vi "Code 0.0.6.vi"(0 "Value":refnum<k5>, 1 "status":bool, 3 "File Path Control":path=path "C:/Projects/FlashProgrammer/RayonM1_01.87.01.txt", 5 "Port":u16=8030, 9 "Drv":u8(ring)=1 items=["Drv 1", "Drv 2"], 11 "error in (no error)":errorcluster) -> (4 "Error List":string, 6 "Status":bool, 15 "error out":errorcluster)   [LabVIEW 2017]
panel:
  out "Array":u16[][](array[numeric])
  out "error out 2":errorcluster
  in  "Delay between sub packets":dbl=0.01 format="%#_13g"
  in  "sub packet Data Length":i32=64
  in  "stop":bool
  out "Time Elapsed":dbl
  in  "MaxSlide":dbl
  out "Autobaud":bool
  in  "StopS.M. 2":bool
  in  "StopS.M.":bool
  in  "CatchNetworkFlag":bool
  in  "stop Listen":bool
  out "conn ID":refnum<k5>
  in  "Next Button":bool
  out "CheckSum":bool[][](array[boolean])
  out "CheckSum DataB":u16 format="%.0x"
  out "CheckSum Data":u16 format="%.0x"
  out "Writting Data":bool
  out "Send Header":bool
  out "sumHeader":u16 format="%.0x"
  # "Ver 0.0.7"
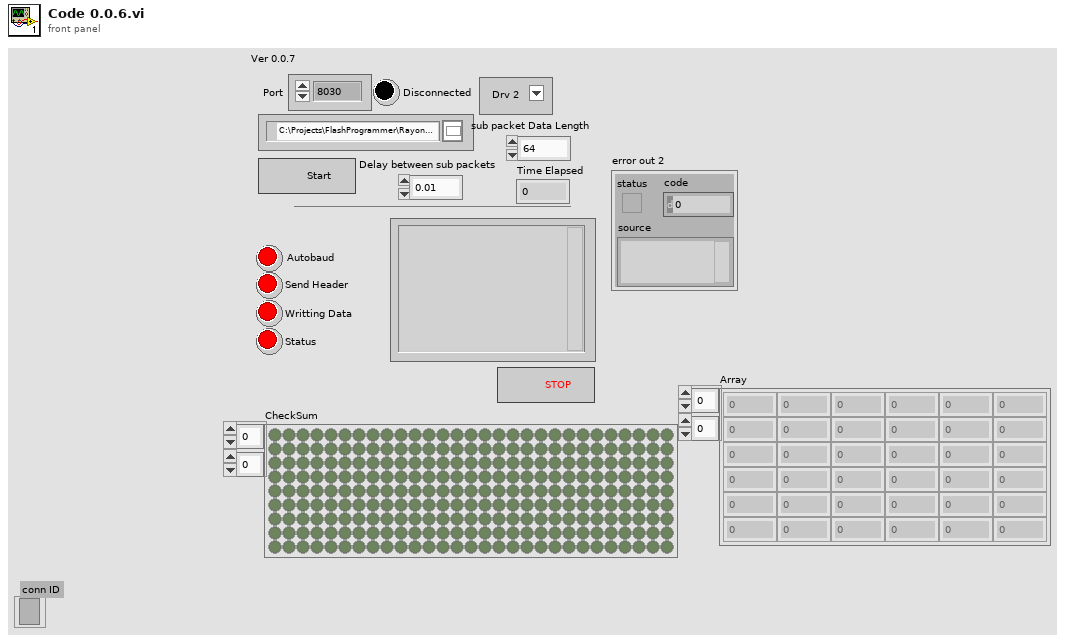
[diagram p1: front panel]
types:
  T1 = enum16{"open", "replace", "create", "open or create", "replace or create", "replace or create with confirmation"}
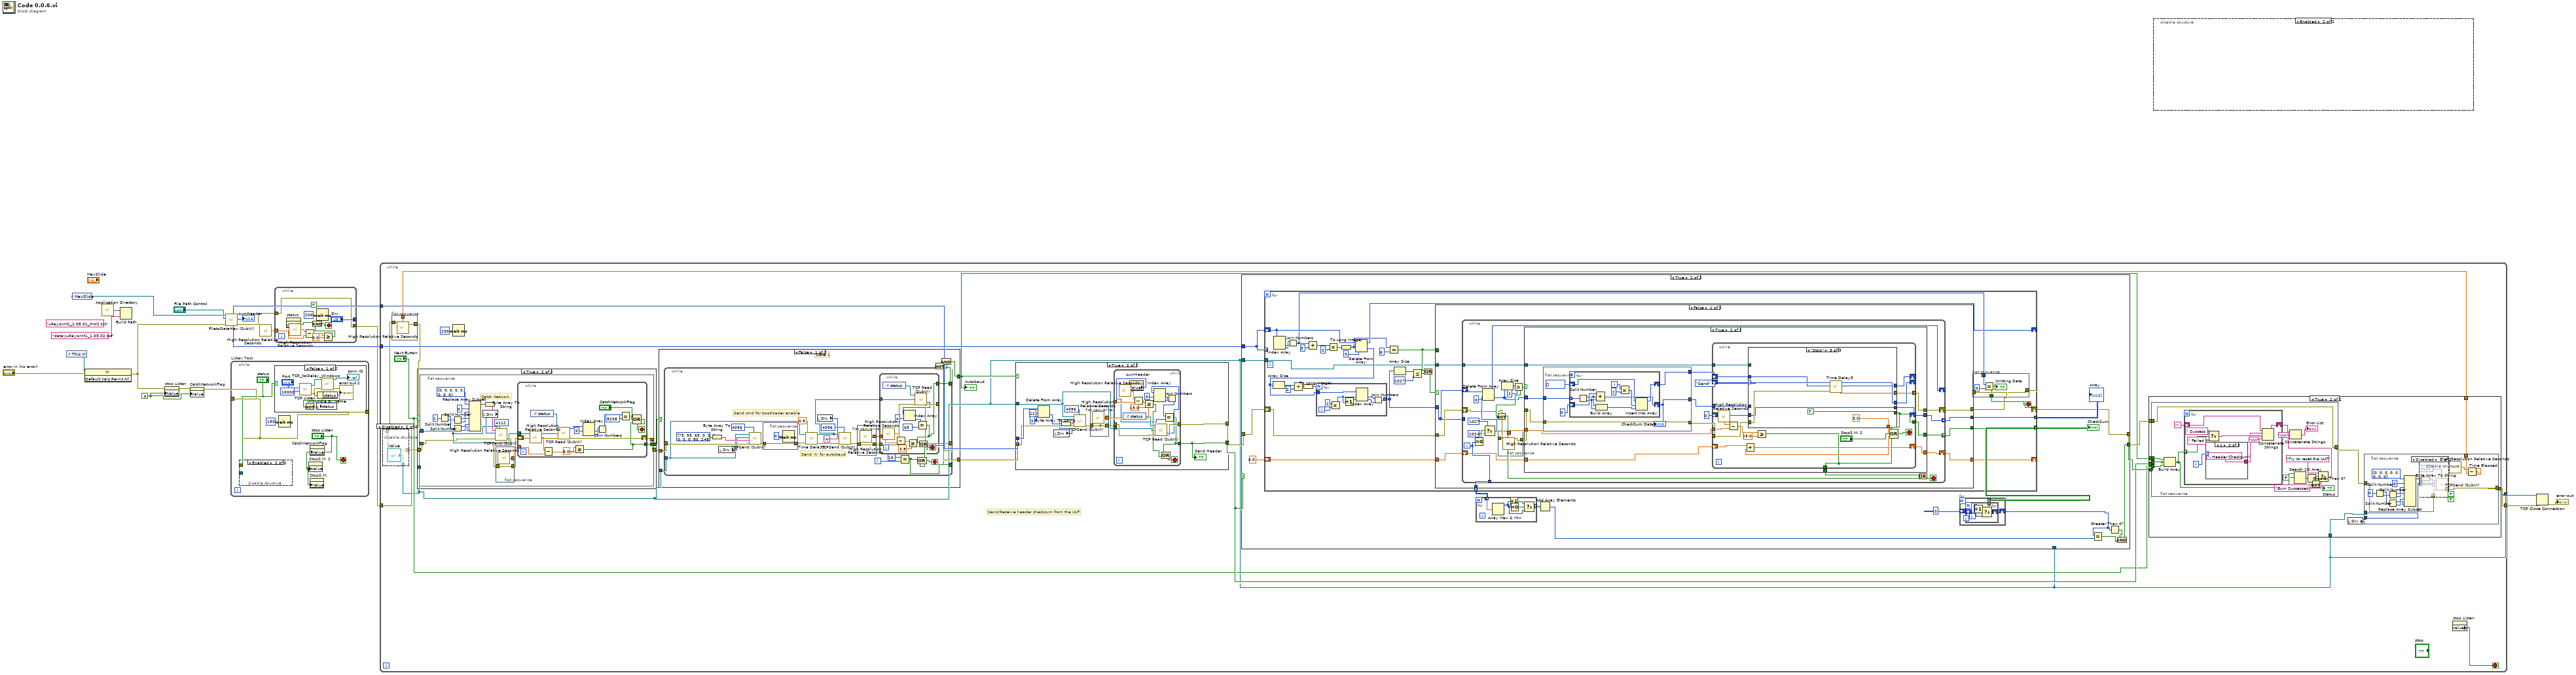
[diagram p0: block diagram]
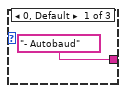
[diagram p4: hidden frame]
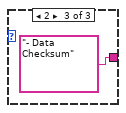
[diagram p5: hidden frame]
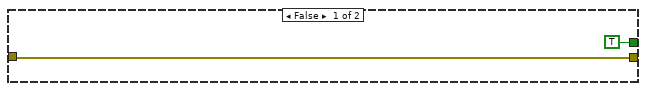
[diagram p6: hidden frame]
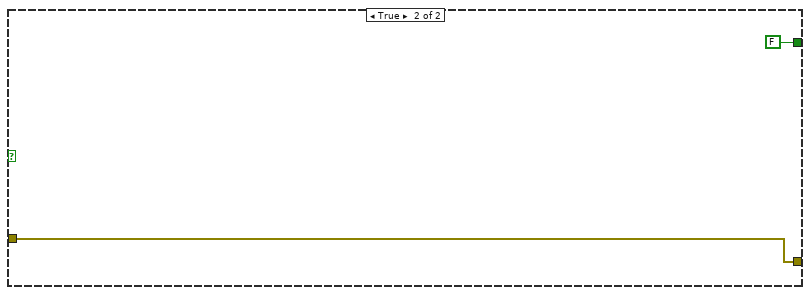
[diagram p7: hidden frame]
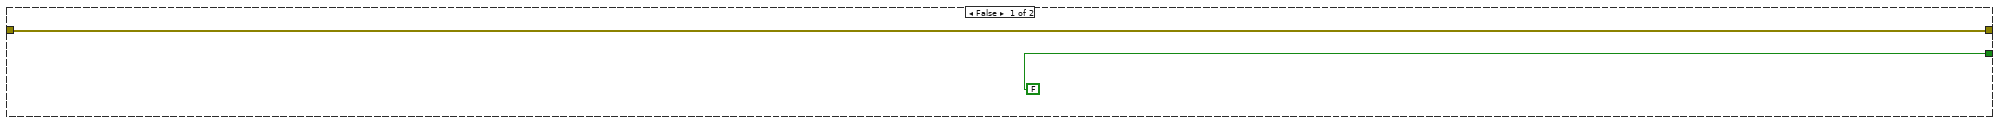
[diagram p8: hidden frame]
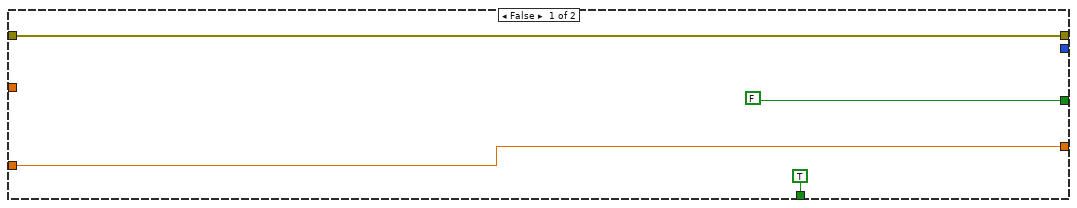
[diagram p9: hidden frame]
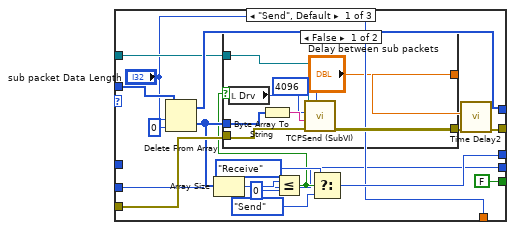
[diagram p10: hidden frame]
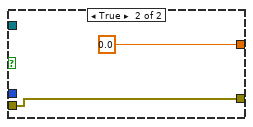
[diagram p11: hidden frame]
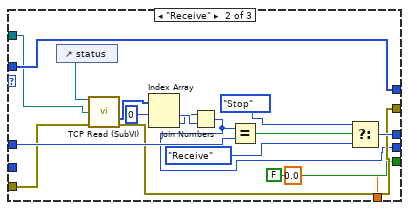
[diagram p12: hidden frame]
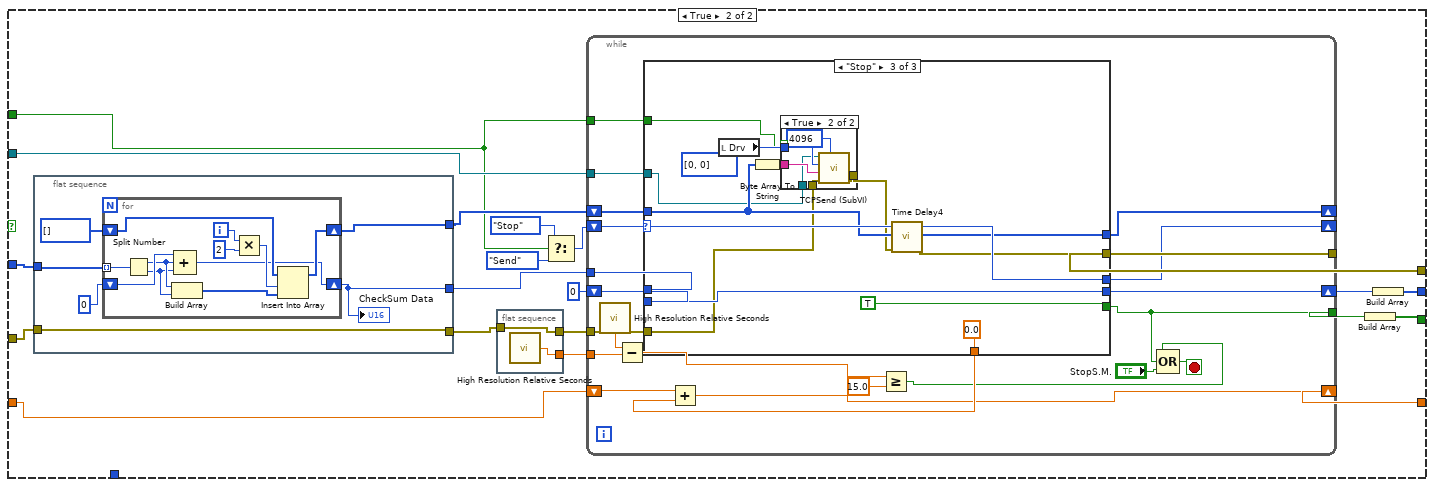
[diagram p13: hidden frame]
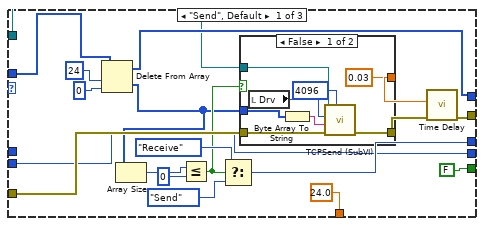
[diagram p14: hidden frame]
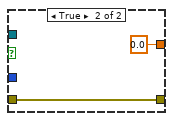
[diagram p15: hidden frame]
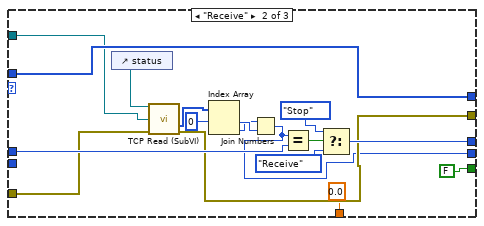
[diagram p16: hidden frame]
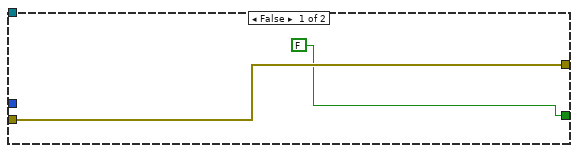
[diagram p18: hidden frame]
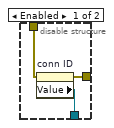
[diagram p19: hidden frame]
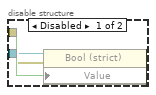
[diagram p20: hidden frame]
diagram:
  (unwired) "uRayonM1_1.05.01_HW2.txt" ("name or relative path")
  w7 = FALSE ("stop")
  n1 = control-ref of="This VI"() -> (w5:refnum<vi>)
  n2 = control-ref of="MaxSlide"() -> (w6:refnum<vi>)
  n3 = invoke class="VI" method="Default Vals.Reinit All"(reference=w5, error in="error in (no error)") -> (error out=w9:errorcluster)  [unwired: 1 in, 2 out]
  n4 = call <vilib>:"Application Directory.vi"() -> ("Application Directory"=w13:path)
  n5 = Build Path(base path=w13, name or relative path="data\\uRayonM1_1.03.02.txt") -> ()  [unwired: 1 out]
  n6 = property on="stop Listen" class="Bool (strict)"(error in=w9, "Value"=w7) -> (error out=w8:errorcluster)  [unwired: 1 in, 1 out]
  n7 = property on="CatchNetworkFlag" class="Bool (strict)"(error in=w8, "Value"=w7) -> (error out=w12:errorcluster)  [unwired: 1 in, 1 out]
  n8 = call "FiletoDataHex (SubVI).vi"("error constant"=w9, "file path (use dialog)"="File Path Control", "Progress bar Max"=w6) -> ("error constant 2"=w4:errorcluster, "Array 2"=w19:u8[], "Array"=w17:u8[], "sumHeader"=→"sumHeader":u16)  [unwired: 2 in, 3 out]
  n9 = while "Listen Task" {
    tunnel: w12 -> [w21]
    tunnel: [w21] -> _
    stop <- "stop Listen" stop-if-true
    n10 = disable-structure shown="Enabled" {
      disable-tunnel: "status" -> [w26 _]
      disable-tunnel: w21 -> [w25 _]
      disable-tunnel: _ -> [w24 _]
      frame Disabled {
        n11 = property class="Bool (strict)"(reference=w24, error in=w25, "Value"=w26) -> ()  [unwired: 2 out]
      }
      frame Enabled {
      }
    }
    n12 = case shown="False" "status" {
      selector: "status" -> [_ w35]
      frame False {
        n13 = call <vilib>:"TCP Listen.vi"("timeout ms (wait forever: -1)"=10000, "port"="Port") -> ("error out"=w28:errorcluster, "connection ID"=w30:refnum<k5>)  [unwired: 5 in, 3 out]
        n14 = Unbundle By Name(w28) -> ("status"=w31:bool)
        n15 = Not(x=w31) -> (.not. x?=w32:bool)
        n16 = local write "status"(w32) -> ()
        n17 = call "TCP_NoDelay_Windows.vi"("error in (no error)"=w28, "connID"=w30) -> ("error out"=→"error out 2":errorcluster, "connID 2"=→"conn ID":refnum<k5>)  [unwired: 4 in]
      }
      frame True {
        n18 = property on="status" class="Bool (strict)"("Value"=w35) -> ()  [unwired: 2 in, 2 out]
      }
    }
    n19 = Wait (ms)(milliseconds to wait=u32 150) -> ()  [unwired: 1 out]
    n20 = property on="StopS.M. 2" class="Bool (strict)"("Value"="stop Listen") -> ()  [unwired: 2 in, 2 out]
    n21 = property on="StopS.M." class="Bool (strict)"("Value"="stop Listen") -> ()  [unwired: 2 in, 2 out]
    n22 = property on="CatchNetworkFlag" class="Bool (strict)"("Value"="stop Listen") -> ()  [unwired: 2 in, 2 out]
  }
  n23 = call <vilib>:"High Resolution Relative Seconds.vi"() -> ("relative seconds"=w11:dbl)
  n24 = while {
    tunnel: w4 -> [w43]
    tunnel: ["Drv"] -> _
    tunnel: [w43] -> w2
    tunnel: w11 -> [w41]
    stop <- w38 stop-if-true
    (unwired) TRUE
    n25 = property on="status" class="Bool (strict)"() -> ("Value"=w36:bool)  [unwired: 2 in, 2 out]
    n26 = call <vilib>:"High Resolution Relative Seconds.vi"() -> ("relative seconds"=w42:dbl)
    n27 = Subtract(x=w42, y=w41) -> (x-y=w40:dbl)
    n28 = Wait (ms)(milliseconds to wait=u32 200) -> ()  [unwired: 1 out]
    n29 = Greater Or Equal?(x=w40, y=3.0) -> (x >= y?=w37:bool)
    n30 = And(x=w36, y=w37) -> (x .and. y?=w38:bool)
  }
  n31 = while {
    tunnel: w19 -> [w64]
    tunnel: w17 -> [w61]
    tunnel: [w46] -> w3
    tunnel: w2 -> [w52]
    tunnel: [w58] -> w16
    stop <- w49 stop-if-true
    # "Send/Receive header checksum from the UUT"
    n32 = disable-structure shown="Disabled" {
      disable-tunnel: w51 -> [w607 w609]
      disable-tunnel: [w606 w609] -> w54
      disable-tunnel: [w605 "Value"] -> w46
      frame Enabled {
        n33 = property on="conn ID" class="Ref (strict)"(error in=w607) -> (error out=w606:errorcluster, "Value"=w605:refnum<k5>)  [unwired: 1 in, 1 out]
      }
      frame Disabled {
      }
    }
    n34 = flat-sequence {
      tunnel: w52 -> [w174]
      tunnel: [w174] -> _
      tunnel: [w175] -> w50
      tunnel: [w174] -> w51
      frame #0 {
        n35 = call <vilib>:"High Resolution Relative Seconds.vi"() -> ("relative seconds"=w175:dbl)
      }
    }
    n36 = case shown="True" "Next Button" {
      tunnel: [w129 w133] -> w62
      tunnel: w54 -> [w129 w132]
      tunnel: w46 -> [_ w131]
      tunnel: [TRUE ("Time has Elapsed") w130] -> w53
      frame False {
      }
      frame True {
        n37 = flat-sequence {
          tunnel: w131 -> [w139]
          tunnel: [w141] -> w133
          tunnel: w132 -> [w137]
          tunnel: [w138] -> w130
          frame #0 {
            # "Catch Network"
            n38 = Split Number(x=u32 1) -> (hi(x)=w151:u16, lo(x)=w150:u16)
            n39 = Split Number(x=w150) -> (hi(x)=w145:u8, lo(x)=w144:u8)
            n40 = Split Number(x=w151) -> (hi(x)=w143:u8, lo(x)=w142:u8)
            n41 = Replace Array Subset(array=u8[] [0, 0, 0, 0, 0, 0, 0, 0] ("unsigned byte array"), new element #1=w144, index #1=0 ("index"), new element #2=w145, new element #3=w142, new element #4=w143) -> (w146:u8[])  [unwired: 3 in]
            n42 = local read "Drv"() -> (w140:u8)
            n43 = Byte Array To String(unsigned byte array=w146) -> (string=w152:string)
            n44 = call "TCPSend (SubVI).vi"("Opcode"=u32 4112, "error in"=w137, "string"=w152, "Drv"=w140, "connection ID"=w139) -> ("error out"=w134:errorcluster)  [unwired: 6 in]
            n45 = flat-sequence {
              tunnel: w134 -> [w154]
              tunnel: [w155] -> w135
              tunnel: [w154] -> w136
              frame #0 {
                n46 = call <vilib>:"High Resolution Relative Seconds.vi"() -> ("relative seconds"=w155:dbl)
              }
            }
            n47 = while {
              shift-right: [w172] -> w141
              shift-left: w136 -> [w173]
              tunnel: w139 -> [w161]
              tunnel: [w156] -> w138
              tunnel: w135 -> [w159]
              stop <- w167 stop-if-true
              n48 = call <vilib>:"High Resolution Relative Seconds.vi"() -> ("relative seconds"=w160:dbl)
              n49 = control-ref of="status"() -> (w166:refnum<vi>)
              n50 = Subtract(x=w160, y=w159) -> (x-y=w158:dbl)
              n51 = call "TCP Read (SubVI).vi"("Status in"=w166, "Value"=w161, "error in (no error)"=w173) -> ("Rx data tmp"=w165:u8[], "error out"=w172:errorcluster)  [unwired: 2 in, 9 out]
              n52 = Greater Or Equal?(x=w158, y=5.0) -> (x >= y?=w156:bool)
              n53 = Index Array(array=w165, index #1=0 ("index")) -> (element #1=w164:u8, element #2=w163:u8)  [unwired: 1 in]
              n54 = Join Numbers(hi=w163, lo=w164) -> ((hi.lo)=w171:u16)
              n55 = Equal?(x=w171, y=u16 8208) -> (x = y?=w169:bool)
              n56 = Compound Arithmetic op=OR("CatchNetworkFlag", w169, w156) -> (w167:bool)
            }
          }
        }
      }
    }
    n57 = Wait (ms)(milliseconds to wait=u32 200) -> ()  [unwired: 1 out]
    n58 = case shown="False" w53 {
      tunnel: w62 -> [w182 w224]
      tunnel: [w181 w224] -> w59
      tunnel: [w179 FALSE] -> w55
      tunnel: w46 -> [w180 _]
      frame False {
        # "State 1"
        n59 = while {
          tunnel: w182 -> [w199]
          tunnel: [w197] -> w181
          tunnel: w180 -> [w184]
          tunnel: [w187] -> w178
          tunnel: [w183] -> w177
          i -> [w203]
          stop <- w204 stop-if-true
          # "Send 'A' for autobaud"
          # "Send cmd for bootloader enable"
          n60 = Byte Array To String(unsigned byte array=u8[] [73, 93, 65, 0, 0, 1, 0, 0, 0, 80, 248] ("output array")) -> (string=w193:string)
          n61 = local read "Drv"() -> (w188:u8)
          n62 = call "TCPSend (SubVI).vi"("Opcode"=u32 4096, "error in"=w199, "string"=w193, "Drv"=w188, "connection ID"=w184) -> ("error out"=w195:errorcluster)  [unwired: 6 in]
          n63 = flat-sequence {
            tunnel: w195 -> [w205]
            tunnel: [w205] -> w194
            frame #0 {
              n64 = Wait (ms)(milliseconds to wait=u32 0) -> ()  [unwired: 1 out]
            }
          }
          n65 = call "Time Delay3"("error in (no error)"=w194, "Delay Time (s)"=0.5) -> ("error out"=w186:errorcluster)  [unwired: 9 in]
          n66 = local read "Drv"() -> (w189:u8)
          n67 = call "TCPSend (SubVI).vi"("Opcode"=u32 4096, "error in"=w186, "string"="A" ("write buffer"), "Drv"=w189, "connection ID"=w184) -> ("error out"=w198:errorcluster)  [unwired: 6 in]
          n68 = flat-sequence {
            tunnel: w198 -> [w208]
            tunnel: [w208] -> w201
            tunnel: [w207] -> w200
            frame #0 {
              n69 = call <vilib>:"High Resolution Relative Seconds.vi"() -> ("relative seconds"=w207:dbl)
            }
          }
          n70 = while {
            tunnel: w201 -> [w213]
            tunnel: w200 -> [w219]
            tunnel: [w212] -> w197
            tunnel: [w210] -> w187
            tunnel: w184 -> [w209]
            stop <- w211 stop-if-true
            n71 = control-ref of="status"() -> (w223:refnum<vi>)
            n72 = call <vilib>:"High Resolution Relative Seconds.vi"() -> ("relative seconds"=w220:dbl)
            n73 = Subtract(x=w220, y=w219) -> (x-y=w218:dbl)
            n74 = Greater Or Equal?(x=w218, y=0.5) -> (x >= y?=w216:bool)
            n75 = call "TCP Read (SubVI).vi"("Status in"=w223, "Value"=w209, "error in (no error)"=w213) -> ("Drv Array"=w221:u8[], "error out"=w212:errorcluster)  [unwired: 2 in, 9 out]
            n76 = Index Array(array=w221, index=0) -> (element=w215:u8)
            n77 = Equal?(x=w215, y=u8 65) -> (x = y?=w210:bool)
            n78 = Or(x=w210, y=w216) -> (x .or. y?=w211:bool)
          }
          n79 = Equal?(x=10, y=w203) -> (x = y?=w183:bool)
          n80 = Compound Arithmetic op=OR(w183, w187) -> (w204:bool)
        }
        n81 = Not(x=w177) -> (.not. x?=w176:bool)
        n82 = And(x=w178, y=w176) -> (x .and. y?=w179:bool)
      }
      frame True {
      }
    }
    "Autobaud" <- w55
    n83 = case shown="True" w55 {
      tunnel: w59 -> [w571 w583]
      tunnel: [w571 w585] -> w57
      tunnel: w61 -> [_ w584]
      tunnel: [FALSE w574] -> w56
      tunnel: w46 -> [_ w572]
      frame False {
      }
      frame True {
        n84 = Delete From Array(array=w584, length=22, index=0) -> (deleted portion=w579:u8[])  [unwired: 1 out]
        n85 = local read "Drv"() -> (w573:u8)
        n86 = Byte Array To String(unsigned byte array=w579) -> (string=w577:string)
        n87 = call "TCPSend (SubVI).vi"("Opcode"=u32 4096, "error in"=w583, "string"=w577, "Drv"=w573, "connection ID"=w572) -> ("error out"=w582:errorcluster)  [unwired: 6 in]
        n88 = flat-sequence {
          tunnel: w582 -> [w586]
          tunnel: [w586] -> _
          tunnel: [w587] -> w575
          tunnel: [w586] -> w576
          frame #0 {
            n89 = call <vilib>:"High Resolution Relative Seconds.vi"() -> ("relative seconds"=w587:dbl)
          }
        }
        n90 = while {
          tunnel: w576 -> [w599]
          tunnel: [w598] -> w585
          tunnel: w575 -> [w603]
          tunnel: [w589] -> w574
          tunnel: w572 -> [w588]
          stop <- w595 stop-if-true
          n91 = call <vilib>:"High Resolution Relative Seconds.vi"() -> ("relative seconds"=w604:dbl)
          n92 = control-ref of="status"() -> (w600:refnum<vi>)
          n93 = property on="sumHeader" class="DigNum (strict)"() -> ("Value"=w590:u16)  [unwired: 2 in, 2 out]
          n94 = Subtract(x=w604, y=w603) -> (x-y=w602:dbl)
          n95 = Greater Or Equal?(x=w602, y=15.0) -> (x >= y?=w594:bool)
          n96 = call "TCP Read (SubVI).vi"("Status in"=w600, "Value"=w588, "error in (no error)"=w599) -> ("Drv Array"=w596:u8[], "error out"=w598:errorcluster)  [unwired: 2 in, 9 out]
          n97 = Index Array(array=w596, index #1=0 ("index")) -> (element #1=w592:u8, element #2=w593:u8)  [unwired: 1 in]
          n98 = Join Numbers(hi=w593, lo=w592) -> ((hi.lo)=w591:u16)
          n99 = Equal?(x=w591, y=w590) -> (x = y?=w589:bool)
          n100 = Compound Arithmetic op=OR(w589, w594) -> (w595:bool)
        }
        "Send Header" <- w574
      }
    }
    n101 = case shown="True" w56 {
      tunnel: w57 -> [w226 w241]
      tunnel: [w226 w228] -> w60
      tunnel: w64 -> [_ w242]
      tunnel: [FALSE w232] -> w63
      tunnel: w46 -> [_ w231]
      tunnel: w46 -> [_ _]
      frame False {
      }
      frame True {
        n102 = for {
          shift-right: [w279] -> _
          shift-left: w242 -> [w287]
          tunnel: w242 -> [_] mode=indexing
          tunnel: [w268] -> w238 mode=indexing
          shift-right: [w255] -> w228
          shift-left: w241 -> [w264]
          tunnel: [w263] -> w240 mode=indexing
          tunnel: w231 -> [w262]
          shift-right: [w260] -> _
          shift-left: 0.0 -> [w261]
          tunnel: [w259] -> w229 mode=indexing
          stop <- w257 stop-if-true
          n103 = Index Array(array=w287) -> (element #1=w286:u8, element #2=w285:u8)  [unwired: 2 in]
          n104 = Join Numbers(hi=w285, lo=w286) -> ((hi.lo)=w258:u16)
          n105 = Add(x=w258, y=u32 3) -> (x+y=w283:u32)
          n106 = Multiply(x=w283, y=u32 2) -> (x*y=w281:u32)
          n107 = To Long Integer(number=w281) -> (32bit integer=w266:i32)
          n108 = Delete From Array(array=w287, length=w266, index=0) -> (deleted portion=w267:u8[], array with subset deleted=w279:u8[])
          n109 = Array Size(array=w267) -> (size(s)=w276:i32)
          n110 = Divide(x=w276, y=2) -> (x/y=w278:dbl)
          n111 = To Long Integer(number=w278) -> (32bit integer=w275:i32)
          n112 = for {
            N: w275 -> [_]
            tunnel: w267 -> [w566]
            tunnel: [w562] -> w272 mode=indexing
            i -> [w565]
            n113 = Multiply(x=2, y=w565) -> (x*y=w568:i32)
            n114 = Increment(x=w568) -> (x+1=w569:i32)
            n115 = Index Array(array=w566, index #1=w568, index #2=w569) -> (element #1=w564:u8, element #2=w563:u8)
            n116 = Join Numbers(hi=w564, lo=w563) -> ((hi.lo)=w562:u16)
          }
          n117 = Equal?(x=w266, y=6) -> (x = y?=w265:bool)
          n118 = Array Size(array=w272) -> (size(s)=w274:i32)
          n119 = Less Or Equal?(x=w274, y=1027) -> (x <= y?=w270:bool)
          n120 = Or(x=w265, y=w270) -> (x .or. y?=w269:bool)
          n121 = case shown="False" w269 {
            tunnel: w264 -> [w299 w453]
            tunnel: [w300 w451] -> w256
            tunnel: w272 -> [w297 w455]
            tunnel: [w298 w454] -> w268
            tunnel: w265 -> [_ w436]
            tunnel: [w296 _] -> w263
            tunnel: w262 -> [w295 w445]
            tunnel: w261 -> [w294 w444]
            tunnel: [w293 w443] -> w260
            tunnel: [w292 w438] -> w259
            frame False {
              n122 = while {
                tunnel: w297 -> [_]
                tunnel: [w312] -> w298 mode=indexing
                shift-right: [w324] -> w300
                shift-left: w299 -> [w303]
                shift-right: [w317] -> _
                shift-left: w297 -> [w323]
                tunnel: [w310] -> w296 mode=indexing
                tunnel: w295 -> [w309]
                shift-right: [w307] -> w293
                shift-left: w294 -> [w308]
                tunnel: [w301] -> w292 mode=indexing
                i -> [w310]
                stop <- w306 stop-if-true
                n123 = Equal To 0?(x=w310) -> (x = 0?=w316:bool)
                n124 = Select(t=1027 ("length"), s=w316, f=1024 ("length")) -> (s? t:f=w313:i32)
                n125 = Delete From Array(array=w323, length=w313, index=0) -> (deleted portion=w311:u16[], array with subset deleted=w317:u16[])
                n126 = flat-sequence {
                  tunnel: w303 -> [w326]
                  tunnel: [w326] -> w302
                  tunnel: [w325] -> w304
                  frame #0 {
                    n127 = call <vilib>:"High Resolution Relative Seconds.vi"() -> ("relative seconds"=w325:dbl)
                  }
                }
                n128 = Array Size(array=w311) -> (size(s)=w321:i32)
                n129 = Greater?(x=w321, y=1) -> (0:w319:bool)
                n130 = Not(x=w319) -> (.not. x?=w318:bool)
                n131 = case shown="True" w319 {
                  tunnel: [w330 w342] -> w324
                  tunnel: w302 -> [w330 w344]
                  tunnel: [FALSE w340] -> w312
                  tunnel: w311 -> [_ w345]
                  tunnel: w309 -> [_ w338]
                  tunnel: w308 -> [w328 w337]
                  tunnel: [w328 w336] -> w307
                  tunnel: [TRUE ("Time has Elapsed") w335] -> w305
                  tunnel: w304 -> [_ w334]
                  tunnel: [_ w332] -> w301
                  frame False {
                  }
                  frame True {
                    n132 = flat-sequence {
                      tunnel: w344 -> [w420]
                      tunnel: [w422] -> w339
                      tunnel: [w419] -> w341
                      tunnel: w345 -> [w421]
                      tunnel: [w420] -> w333
                      frame #0 {
                        n133 = for {
                          tunnel: w421 -> [w435] mode=indexing
                          shift-right: [w430] -> w422
                          shift-left: u8[] [] -> [w429]
                          shift-right: [w427] -> w419
                          shift-left: u16 0 -> [w428]
                          i -> [w434]
                          n134 = Split Number(x=w435) -> (hi(x)=w426:u8, lo(x)=w425:u8)
                          n135 = Build Array(w426, w425) -> (w432:u8[])
                          n136 = Compound Arithmetic op=ADD(w428, w426, w425) -> (w427:u16)
                          n137 = Multiply(x=w434, y=2) -> (x*y=w431:i32)
                          n138 = Insert Into Array(array=w429, index=w431, new element=w432) -> (w430:u8[])
                        }
                        "CheckSum DataB" <- w419
                      }
                    }
                    n139 = while {
                      shift-right: [w364] -> _
                      shift-left: enum16{"Stop", "Receive", "Send"}."Send" -> [w366]
                      shift-right: [w362] -> _
                      shift-left: w339 -> [w365]
                      tunnel: w341 -> [w363]
                      tunnel: [w358] -> w340
                      tunnel: [w361] -> w342
                      tunnel: w338 -> [w357]
                      shift-right: [w354] -> w336
                      shift-left: w337 -> [w356]
                      tunnel: [w349] -> w335
                      tunnel: w333 -> [w353]
                      tunnel: w334 -> [w348]
                      shift-right: [w347] -> w332
                      shift-left: u16 0 -> [w346]
                      stop <- w360 stop-if-true
                      n140 = call <vilib>:"High Resolution Relative Seconds.vi"() -> ("relative seconds"=w352:dbl)
                      n141 = Subtract(x=w352, y=w348) -> (x-y=w351:dbl)
                      n142 = case shown="\"Stop\"" w366 {
                        selector: w366 -> [_ _ w418]
                        tunnel: w365 -> [w383 w402 w416]
                        tunnel: [w380 w404 w418] -> w364
                        tunnel: w353 -> [w379 w400 w415]
                        tunnel: w363 -> [_ w406 _]
                        tunnel: [FALSE FALSE TRUE] -> w358
                        tunnel: [w375 w402 w416] -> w362
                        tunnel: [w373 w401 w412] -> w361
                        tunnel: w357 -> [w369 w397 _]
                        tunnel: ["sub packet Data Length" 0.0 ("y") 0.0 ("y")] -> w355
                        tunnel: [w367 w395 w413] -> w347
                        tunnel: w346 -> [w367 _ w413]
                        frame "Send", Default {
                          n143 = Delete From Array(array=w383, length="sub packet Data Length", index=0) -> (deleted portion=w372:u8[], array with subset deleted=w375:u8[])
                          n144 = Array Size(array=w372) -> (size(s)=w381:i32)
                          n145 = Less Or Equal?(x=w381, y=0) -> (x <= y?=w371:bool)
                          n146 = case shown="False" w371 {
                            tunnel: w372 -> [w389 _]
                            tunnel: w379 -> [w388 w394]
                            tunnel: [w387 w394] -> w374
                            tunnel: ["Delay between sub packets" 0.0 ("Delay Time (s)")] -> w370
                            tunnel: w369 -> [w385 _]
                            frame False {
                              n147 = local read "Drv"() -> (w390:u8)
                              n148 = Byte Array To String(unsigned byte array=w389) -> (string=w391:string)
                              n149 = call "TCPSend (SubVI).vi"("Opcode"=u32 4096, "error in"=w388, "string"=w391, "Drv"=w390, "connection ID"=w385) -> ("error out"=w387:errorcluster)  [unwired: 6 in]
                            }
                            frame True {
                            }
                          }
                          n150 = Select(t=enum16{"Stop", "Receive", "Send"}."Receive", s=w371, f=enum16{"Stop", "Receive", "Send"}."Send") -> (s? t:f=w380:enum16{"Stop", "Receive", "Send"})
                          n151 = call "Time Delay2"("error in (no error)"=w374, "Delay Time (s)"=w370) -> ("error out"=w373:errorcluster)  [unwired: 9 in]
                        }
                        frame "Receive" {
                          n152 = control-ref of="status"() -> (w411:refnum<vi>)
                          n153 = call "TCP Read (SubVI).vi"("Status in"=w411, "Value"=w397, "error in (no error)"=w400) -> ("Drv Array"=w407:u8[], "error out"=w401:errorcluster)  [unwired: 2 in, 9 out]
                          n154 = Index Array(array=w407, index #1=0 ("index")) -> (element #1=w410:u8, element #2=w409:u8)  [unwired: 1 in]
                          n155 = Join Numbers(hi=w409, lo=w410) -> ((hi.lo)=w395:u16)
                          n156 = Equal?(x=w395, y=w406) -> (x = y?=w399:bool)
                          n157 = Select(t=enum16{"Stop", "Receive", "Send"}."Stop", s=w399, f=enum16{"Stop", "Receive", "Send"}."Receive") -> (s? t:f=w404:enum16{"Stop", "Receive", "Send"})
                        }
                        frame "Stop" {
                          n158 = call "Time Delay5"("error in (no error)"=w415) -> ("error out"=w412:errorcluster)  [unwired: 10 in]
                        }
                      }
                      n159 = Add(x=w356, y=w355) -> (x+y=w354:dbl)
                      n160 = Greater Or Equal?(x=w351, y=15.0) -> (x >= y?=w349:bool)
                      n161 = Compound Arithmetic op=OR(w358, "StopS.M. 2", w349) -> (w360:bool)
                    }
                  }
                }
                n162 = Or(x=w305, y=w318) -> (x .or. y?=w306:bool)
              }
            }
            frame True {
              n163 = flat-sequence {
                tunnel: w453 -> [w546]
                tunnel: [w548] -> w446
                tunnel: w455 -> [w547]
                tunnel: [w546] -> w442
                tunnel: [w545] -> w452
                frame #0 {
                  n164 = for {
                    tunnel: w547 -> [w561] mode=indexing
                    shift-right: [w556] -> w548
                    shift-left: u8[] [] -> [w555]
                    shift-right: [w553] -> w545
                    shift-left: u16 0 -> [w554]
                    i -> [w560]
                    n165 = Split Number(x=w561) -> (hi(x)=w552:u8, lo(x)=w551:u8)
                    n166 = Build Array(w552, w551) -> (w558:u8[])
                    n167 = Compound Arithmetic op=ADD(w554, w552, w551) -> (w553:u16)
                    n168 = Multiply(x=w560, y=2) -> (x*y=w557:i32)
                    n169 = Insert Into Array(array=w555, index=w557, new element=w558) -> (w556:u8[])
                  }
                  "CheckSum Data" <- w545
                }
              }
              n170 = flat-sequence {
                tunnel: w442 -> [w457]
                tunnel: [w457] -> w441
                tunnel: [w456] -> w440
                frame #0 {
                  n171 = call <vilib>:"High Resolution Relative Seconds.vi"() -> ("relative seconds"=w456:dbl)
                }
              }
              n172 = Select(t=enum16{"Stop", "Receive", "Send"}."Stop", s=w436, f=enum16{"Stop", "Receive", "Send"}."Send") -> (s? t:f=w449:enum16{"Stop", "Receive", "Send"})
              n173 = while {
                shift-right: [w477] -> _
                shift-left: w449 -> [w479]
                shift-right: [w475] -> _
                shift-left: w446 -> [w478]
                tunnel: w441 -> [w468]
                tunnel: w452 -> [w476]
                tunnel: [w474] -> w447
                tunnel: [w473] -> w451
                tunnel: w445 -> [w470]
                shift-right: [w466] -> w443
                shift-left: w444 -> [w469]
                tunnel: w440 -> [w465]
                shift-right: [w460] -> w439
                shift-left: u16 0 -> [w459]
                tunnel: w436 -> [w458]
                stop <- w472 stop-if-true
                n174 = call <vilib>:"High Resolution Relative Seconds.vi"() -> ("relative seconds"=w464:dbl)
                n175 = Subtract(x=w464, y=w465) -> (x-y=w463:dbl)
                n176 = case shown="\"Stop\"" w479 {
                  selector: w479 -> [_ _ w537]
                  tunnel: w478 -> [w482 w515 w530]
                  tunnel: [w496 w517 w537] -> w477
                  tunnel: w468 -> [w495 w513 w529]
                  tunnel: w476 -> [_ w520 _]
                  tunnel: [FALSE FALSE TRUE] -> w474
                  tunnel: [w491 w515 w530] -> w475
                  tunnel: [w489 w514 w533] -> w473
                  tunnel: w470 -> [w487 w511 w526]
                  tunnel: [24.0 ("x") 0.0 ("x") 0.0 ("x")] -> w467
                  tunnel: [w485 w509 w534] -> w460
                  tunnel: w459 -> [w485 _ w534]
                  tunnel: w458 -> [_ _ w527]
                  frame "Send", Default {
                    n177 = Delete From Array(array=w482, length=24, index=0) -> (deleted portion=w483:u8[], array with subset deleted=w491:u8[])
                    n178 = Array Size(array=w483) -> (size(s)=w497:i32)
                    n179 = Less Or Equal?(x=w497, y=0) -> (x <= y?=w484:bool)
                    n180 = Select(t=enum16{"Stop", "Receive", "Send"}."Receive", s=w484, f=enum16{"Stop", "Receive", "Send"}."Send") -> (s? t:f=w496:enum16{"Stop", "Receive", "Send"})
                    n181 = case shown="False" w484 {
                      tunnel: w483 -> [w503 _]
                      tunnel: w495 -> [w502 w508]
                      tunnel: [w501 w508] -> w490
                      tunnel: [0.03 ("Delay Time (s)") 0.0 ("Delay Time (s)")] -> w488
                      tunnel: w487 -> [w499 _]
                      frame False {
                        n182 = local read "Drv"() -> (w504:u8)
                        n183 = Byte Array To String(unsigned byte array=w503) -> (string=w505:string)
                        n184 = call "TCPSend (SubVI).vi"("Opcode"=u32 4096, "error in"=w502, "string"=w505, "Drv"=w504, "connection ID"=w499) -> ("error out"=w501:errorcluster)  [unwired: 6 in]
                      }
                      frame True {
                      }
                    }
                    n185 = call "Time Delay"("error in (no error)"=w490, "Delay Time (s)"=w488) -> ("error out"=w489:errorcluster)  [unwired: 9 in]
                  }
                  frame "Receive" {
                    n186 = control-ref of="status"() -> (w525:refnum<vi>)
                    n187 = call "TCP Read (SubVI).vi"("Status in"=w525, "Value"=w511, "error in (no error)"=w513) -> ("Drv Array"=w521:u8[], "error out"=w514:errorcluster)  [unwired: 2 in, 9 out]
                    n188 = Index Array(array=w521, index #1=0 ("index")) -> (element #1=w524:u8, element #2=w523:u8)  [unwired: 1 in]
                    n189 = Join Numbers(hi=w523, lo=w524) -> ((hi.lo)=w509:u16)
                    n190 = Equal?(x=w509, y=w520) -> (x = y?=w519:bool)
                    n191 = Select(t=enum16{"Stop", "Receive", "Send"}."Stop", s=w519, f=enum16{"Stop", "Receive", "Send"}."Receive") -> (s? t:f=w517:enum16{"Stop", "Receive", "Send"})
                  }
                  frame "Stop" {
                    (unwired) u8[] [0, 0] ("unsigned byte array")
                    n192 = local read "Drv"() -> (w531:u8)
                    n193 = Byte Array To String(unsigned byte array=w530) -> (string=w532:string)
                    n194 = case shown="True" w527 {
                      tunnel: w532 -> [_ w544]
                      tunnel: w531 -> [_ w543]
                      tunnel: w529 -> [w538 w541]
                      tunnel: [w538 w540] -> w528
                      tunnel: w526 -> [_ w539]
                      frame False {
                      }
                      frame True {
                        n195 = call "TCPSend (SubVI).vi"("Opcode"=u32 4096, "error in"=w541, "string"=w544, "Drv"=w543, "connection ID"=w539) -> ("error out"=w540:errorcluster)  [unwired: 6 in]
                      }
                    }
                    n196 = call "Time Delay4"("error in (no error)"=w528) -> ("error out"=w533:errorcluster)  [unwired: 10 in]
                  }
                }
                n197 = Add(x=w469, y=w467) -> (x+y=w466:dbl)
                n198 = Greater Or Equal?(x=w463, y=15.0) -> (x >= y?=w461:bool)
                n199 = Compound Arithmetic op=OR(w461, w474, "StopS.M.") -> (w472:bool)
              }
              n200 = Build Array(w447) -> (w454:bool[])
              n201 = Build Array(w439) -> (w438:u16[])
            }
          }
          n202 = flat-sequence {
            tunnel: w258 -> [w290]
            tunnel: [w289] -> w257
            tunnel: w256 -> [w288]
            tunnel: [w288] -> w255
            frame #0 {
              n203 = Equal?(x=w290, y=u16 0) -> (x = y?=w289:bool)
              "Writting Data" <- w289
            }
          }
        }
        "CheckSum" <- w238
        "Array" <- w229
        n204 = for {
          tunnel: w240 -> [w254] mode=indexing
          tunnel: [w250] -> w239 mode=indexing
          n205 = Array Max & Min(array=w254) -> (max value=w251:i32)  [unwired: 3 out]
          n206 = Increment(x=w251) -> (x+1=w252:i32)
          n207 = Equal To 0?(x=w251) -> (x = 0?=w253:bool)
          n208 = Select(t=w252, s=w253, f=w251) -> (s? t:f=w250:i32)
        }
        n209 = Add Array Elements(numeric array=w239) -> (sum=w236:i32)
        n210 = for {
          tunnel: w238 -> [w245] mode=indexing
          shift-right: [w244] -> w235
          shift-left: 0 -> [w243]
          n211 = for {
            tunnel: w245 -> [w249] mode=indexing
            shift-right: [w247] -> w244
            shift-left: w243 -> [w246]
            n212 = Increment(x=w246) -> (x+1=w248:i32)
            n213 = Select(t=w248, s=w249, f=w246) -> (s? t:f=w247:i32)
          }
        }
        n214 = Equal?(x=w235, y=w236) -> (x = y?=w233:bool)
        n215 = Greater Than 0?(x=w235) -> (x > 0?=w234:bool)
        n216 = And(x=w234, y=w233) -> (x .and. y?=w232:bool)
      }
    }
    n217 = case shown="True" "Next Button" {
      tunnel: w63 -> [_ w74]
      tunnel: w60 -> [w65 w73]
      tunnel: [w65 w71] -> w58
      tunnel: w56 -> [_ w70]
      tunnel: w55 -> [_ w69]
      tunnel: w46 -> [_ w68]
      tunnel: w50 -> [_ w67]
      frame False {
      }
      frame True {
        n218 = flat-sequence {
          tunnel: w73 -> [w115]
          tunnel: [w115] -> w72
          tunnel: w69 -> [w114]
          tunnel: [w102] -> _
          tunnel: w74 -> [w113]
          tunnel: w70 -> [w102]
          frame #0 {
            n219 = Build Array(w114, w102, w113) -> (w108:bool[])
            n220 = for {
              tunnel: w108 -> [w124] mode=indexing
              shift-right: [w122] -> w111
              shift-left: "" -> [w123]
              i -> [w120]
              n221 = case shown="1" w120 {
                tunnel: ["- Autobaud" "- Header Checksum" "- Data Checksum"] -> w119
                frame 0, Default {
                }
                frame 1 {
                }
                frame 2 {
                }
              }
              n222 = Select(t=" Success !", s=w124, f=" Failed !") -> (s? t:f=w118:string)
              n223 = Concatenate Strings(w123, w119, w118, "\r\n") -> (w122:string)
            }
            n224 = Search 1D Array(1D array=w108, element=FALSE) -> (index of element=w106:i32)  [unwired: 1 in]
            n225 = Greater Than 0?(x=w106) -> (x > 0?=w101:bool)
            n226 = Not(x=w101) -> (.not. x?=→"Status":bool)
            n227 = Select(t="Try to reset the UUT" ("string"), s=w101, f="Burn Successed.") -> (s? t:f=w104:string)
            n228 = Concatenate Strings(w111, "\r\n", w104) -> (→"Error List":string)
          }
        }
        n229 = local read "Drv"() -> (w66:u8)
        n230 = flat-sequence {
          tunnel: w72 -> [w92]
          tunnel: w66 -> [w91]
          tunnel: w68 -> [w90]
          tunnel: [w78] -> w71
          tunnel: w67 -> [w76]
          frame #0 {
            (unwired) FALSE ("stop Listen")
            (unwired) TRUE ("stop Listen")
            n231 = Split Number(x=u32 0) -> (hi(x)=w89:u16, lo(x)=w88:u16)
            n232 = Split Number(x=w88) -> (hi(x)=w83:u8, lo(x)=w82:u8)
            n233 = Split Number(x=w89) -> (hi(x)=w81:u8, lo(x)=w80:u8)
            n234 = Replace Array Subset(array=u8[] [0, 0, 0, 0, 0, 0, 0, 0] ("unsigned byte array"), new element #1=w82, index #1=0 ("index"), new element #2=w83, new element #3=w80, new element #4=w81) -> (w84:u8[])  [unwired: 3 in]
            n235 = Byte Array To String(unsigned byte array=w84) -> (string=w79:string)
            n236 = disable-structure shown="Disabled" {
              disable-tunnel: w92 -> [w98 w99]
              disable-tunnel: w91 -> [w97 _]
              disable-tunnel: w90 -> [w96 _]
              disable-tunnel: w79 -> [w94 _]
              disable-tunnel: [w93 w99] -> w78
              frame Disabled {
                n237 = call "TCPSend (SubVI).vi"("Opcode"=u32 4112, "error in"=w98, "string"=w94, "Drv"=w97, "connection ID"=w96) -> ("error out"=w93:errorcluster)  [unwired: 6 in]
              }
              frame Enabled {
              }
            }
            n238 = call <vilib>:"High Resolution Relative Seconds.vi"() -> ("relative seconds"=w77:dbl)
            n239 = Subtract(x=w77, y=w76) -> (x-y=→"Time Elapsed":dbl)
          }
        }
      }
    }
    n240 = property on="stop Listen" class="Bool (strict)"() -> ("Value"=w49:bool)  [unwired: 2 in, 2 out]
  }
  n241 = disable-structure shown="Enabled" {
    frame Disabled {
      n242 = call <vilib>:"Application Directory.vi"() -> ("Application Directory"=w614:path)
      n243 = Build Path(base path=w614, name or relative path="ans.txt") -> (appended path=w613:path)
      n244 = Open/Create/Replace File(file path (use dialog)=w613, operation (0:open)=T1."open or create") -> (refnum out=w610:refnum<file>, error out=w611:errorcluster)  [unwired: 4 in, 1 out]
      n245 = for {
        tunnel: _ -> [w626] mode=indexing
        tunnel: w611 -> [w624]
        tunnel: w610 -> [w623]
        i -> [w619]
        n246 = Quotient & Remainder(x=w619, y=24 ("x")) -> (x-y*floor(x/y)=w617:i32)  [unwired: 1 out]
        n247 = Format Into String(format string="%02x", w626) -> (resulting string=w622:string)  [unwired: 2 in, 1 out]
        n248 = Equal?(x=w617, y=0) -> (x = y?=w620:bool)
        n249 = case shown="True" w620 {
          tunnel: w622 -> [w629 w632]
          tunnel: [w628 w631] -> w621
          frame False {
            n250 = call <vilib>:"Space Constant.vi"() -> ("String"=w627:string)
            n251 = Concatenate Strings(w629, w627) -> (w628:string)
          }
          frame True {
            n252 = Concatenate Strings(w632, "\r\n") -> (w631:string)
          }
        }
        n253 = Write to Text File(file (use dialog)=w623, text=w621, error in=w624) -> ()  [unwired: 1 in, 3 out]
      }
    }
    frame Enabled {
    }
  }
  n254 = TCP Close Connection(connection ID=w3, error in (no error)=w16) -> (error out=→"error out":errorcluster)  [unwired: 1 in, 1 out]
